vi "From JSON Text (LVObject).vi"(7 "Data Type (default value)":refnum<class>, 9 "error in (no error)":errorcluster, 10 "Offset":i32, 11 "JSON":string) -> (1 "error out":errorcluster, 2 "Offset past match":i32, 3 "LabVIEW Object":refnum<class>)   [LabVIEW 2017, in "JSONtext.lvlib"]
doc: "Gets LabVIEW Object that has been flattened and stored as a JSON String."
uses:
  JSONtext.lvlib
  support/Get LVObject.vi
  support/Get String.vi
  Parsing/Advance past String.vi
  String Subset.vi
  support/Strip Quotes and Unescape.vi
  support/Unescape JSON string.vi
  Parsing/Parsing Error.vi
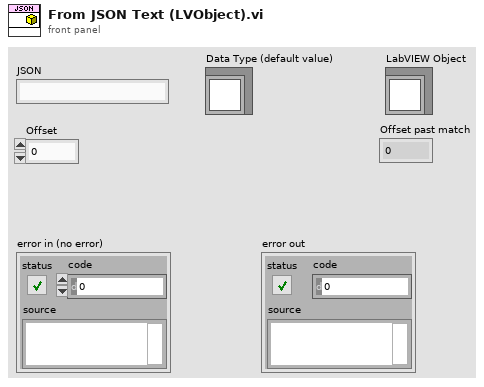
[diagram p1: front panel]
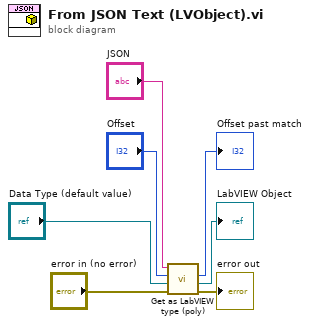
[diagram p0: block diagram]
diagram:
  n1 = call-poly "Get as LabVIEW type (poly).vi"("error in (no error)"="error in (no error)", "Object Type"="Data Type (default value)", "Offset"="Offset", "JSON String containing Flattened Object"="JSON") -> ("error out"=→"error out":errorcluster, "Object out"=→"LabVIEW Object":refnum<class>, "Offset past match"=→"Offset past match":i32)  [unwired: 5 in]
